vi "Measure.vi"(8 "error in (no error)":errorcluster, 9 "measurement configuration":variant, 10 "measure call context in":refnum<class "Measure Call Context.lvclass">, 11 "measurement plugin in":refnum<class "DCPower Single Meas Per Trigger.lvclass">) -> (0 "error out":errorcluster, 1 "measurement results":variant, 2 "measure call context out":refnum<class "Measure Call Context.lvclass">, 3 "measurement plugin out":refnum<class "DCPower Single Meas Per Trigger.lvclass">)   [LabVIEW 2025, in "DCPower Single Meas Per Trigger.lvclass"]
uses:
  DCPower Single Meas Per Trigger.lvclass
  <vilib>/Plug-In SDKs/Measurements/Measure Call Context/Measure Call Context.lvclass
  Measurement Configuration.ctl
  DCPower Single Meas Per Trigger.lvclass/DCPower Single Meas Per Trigger.ctl
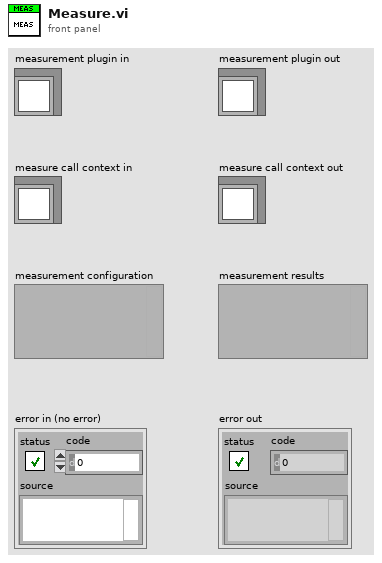
[diagram p1: front panel]
types:
  T1 = typedef "DCPower Single Meas Per Trigger.lvclass/Measurement Configuration.ctl" = cluster{"Resource Name":string, "Measure Trigger Source":string, "Voltage Level":dbl, "Current Limit":dbl, "Aperture Time":dbl, "Current Unit":string, "Delimited Text":string, "Run Until":dbl}
  T2 = typedef "DCPower Single Meas Per Trigger.lvclass/Measurement Results.ctl" = cluster{"Text Result":string, "Measured Voltages":dbl[], "Measured Currents":dbl[]}
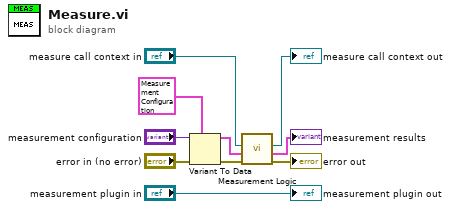
[diagram p0: block diagram]
diagram:
  n1 = Variant To Data(error in="error in (no error)", type=T1 {"Resource Name"="", "Measure Trigger Source"="", "Voltage Level"=64.0, "Current Limit"=32.0, "Aperture Time"=1.2, "Current Unit"="Lorem ipsum dolor sit", "Delimited Text"=",", "Run Until"=inf} ("measurement configuration"), Variant="measurement configuration") -> (data=w1:T1, error out=w7:errorcluster)
  n2 = call "Measurement Logic.vi"("error in"=w7, "measurement configuration"=w1, "measure call context in"="measure call context in") -> ("error out"=→"error out":errorcluster, "measurement results"=→"measurement results":T2, "measure call context out"=→"measure call context out":refnum<class "Measure Call Context.lvclass">)  [unwired: 6 in]
  "measurement plugin out" <- "measurement plugin in"
